vi "ExStreamToFilefNoDisplay.vi"() -> ()   [LabVIEW 2010]
uses:
  Open-Close Hardware/CamHandle.vi
panel:
  out "done collecting":bool
  out "beta":u32
  out "build":u32
  out "Minor":u32
  out "Major":u32
  in  "stop collection 2":bool
  in  "data collection type\n1 - stream to file\n2 - stream to ram, then file":u32=2 min=1 step=1
  in  "stop collection":bool
  in  "Path":path=path "C:/Users/Public/Documents/SItoolkit/LabVIEW/Data Files/nframe"
  in  "Number of Images":u32=50 min=1 step=1
  out "ready to \nstart":bool
  in  "Start collection":bool
  in  "Exposure":dbl=1e-05 min=0.0 step=1e-06 format="%.7f"
  out "error out":errorcluster
  in  "error in (no error)":errorcluster
  # "ExCNframeBigBufNoDisplay:\nThis example collects,  and saves in \na .spe file the number of images selected. This \nexample requires the camera have circular \nbuffers capability. \nFirst this example creates an array of image \nhandles. It then collects data into this array.\nFinally it displays and saves all the images."
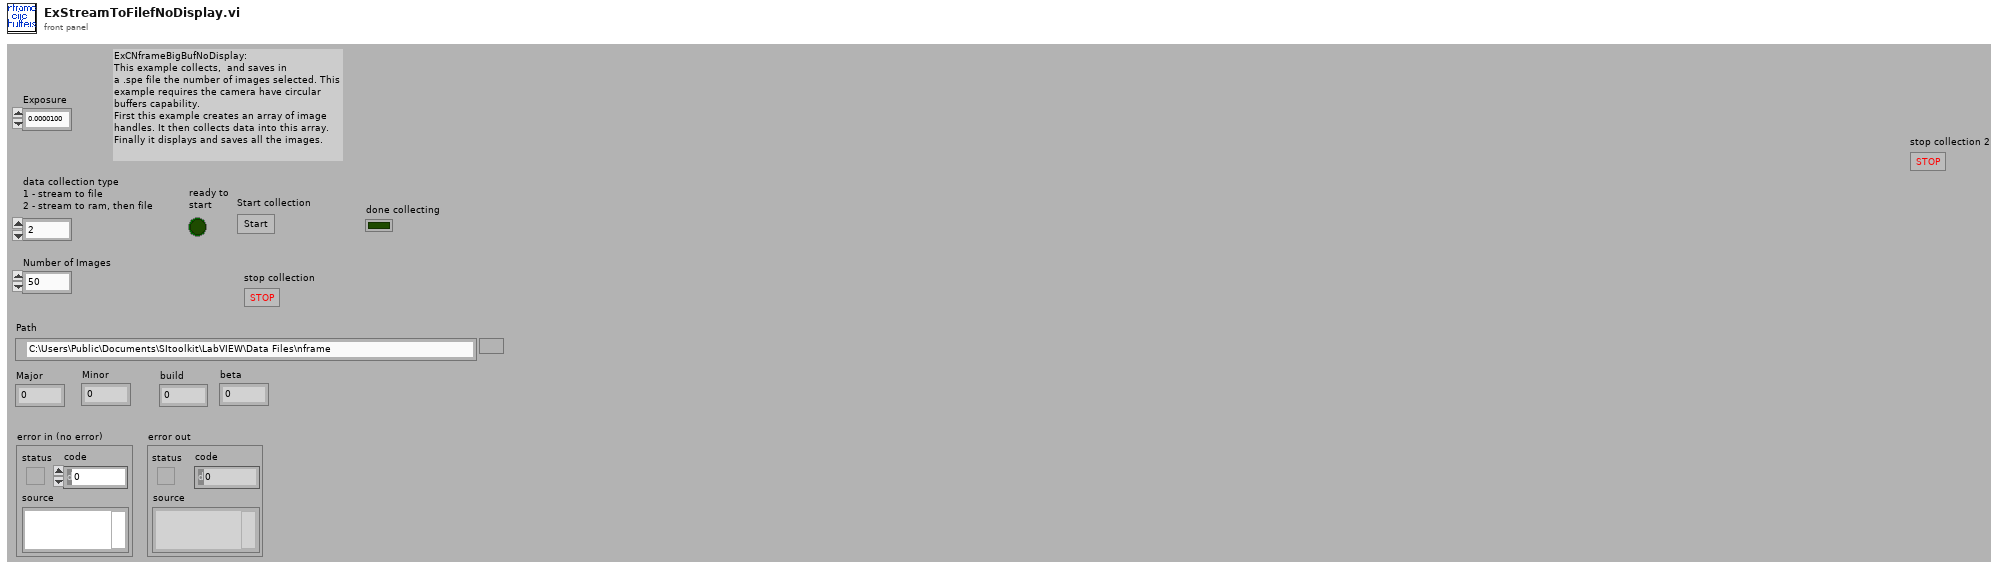
[diagram p1: front panel]
types:
  T1 = cluster{"Major Version":u32, "Minor Version":u32, "External Build":u32, "Internal Build":u32}
  T2 = cluster{"acquire focus mode":u32, "Exposure":dbl, "Number of Images":u32, "Software accumulation":u32}
  T3 = cluster{"Camera Handle":u32, "Pulser Handle":u32, "File Handle":u32, "Display Handle":u32, "Image Handle":u32}
  T4 = cluster{"Exposure":dbl, "acquire focus mode":u32, "Number of Images":u32, "Software accumulation":u32}
  T5 = cluster{"Camera Handle":u32, "File Handle":u32, "Image Handle":u32}
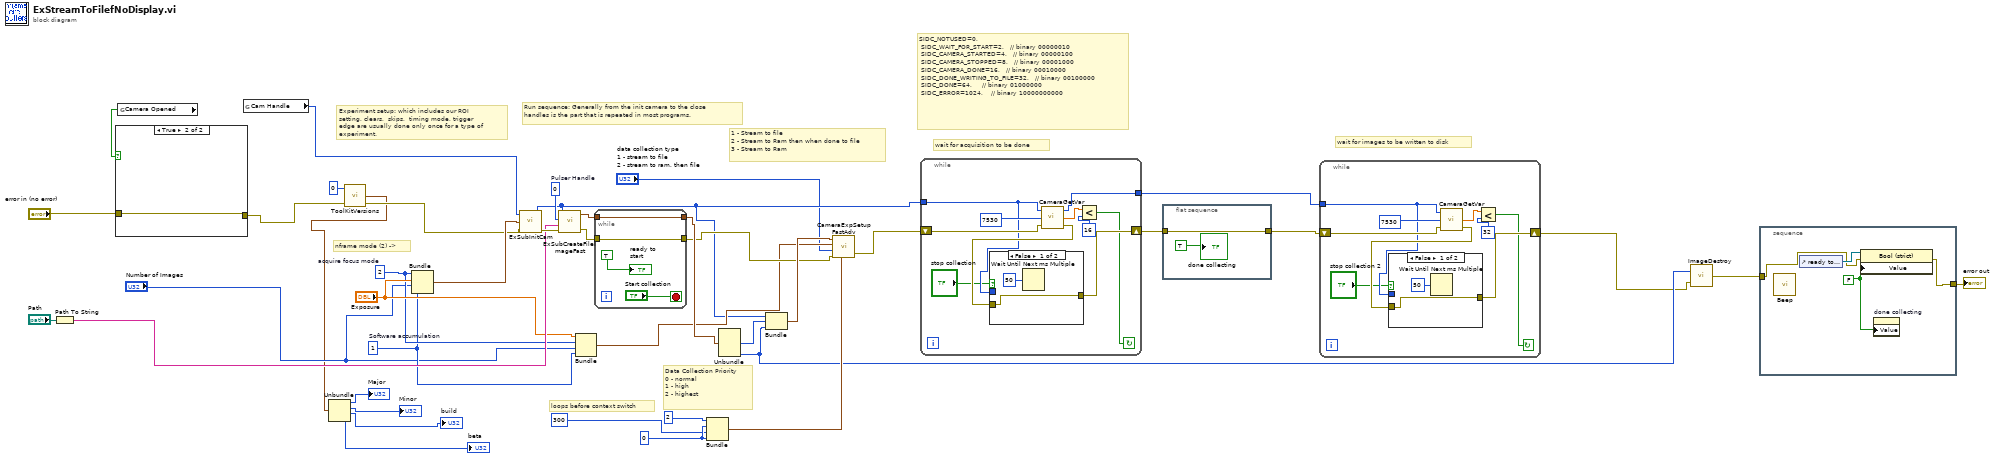
[diagram p0: block diagram]
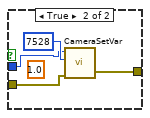
[diagram p2: hidden frame]
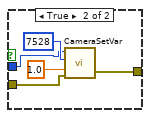
[diagram p3: hidden frame]
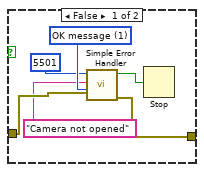
[diagram p4: hidden frame]
diagram:
  w29 = u32 0
  w40 = u32 0  # Pulser Handle
  w26 = u32 2  # acquire focus mode
  w25 = u32 1  # Software accumulation
  # "SIDC_NOTUSED=0,\n\tSIDC_WAIT_FOR_START=2,\t\t\t// binary 00000010\n\tSIDC_CAMERA_STARTED=4,\t\t\t// binary 00000100\n\tSIDC_CAMERA_STOPPED=8,\t\t\t// binary 00001000\n\tSIDC_CAMERA_DONE=16,\t\t\t// binary 00010000\n\tSIDC_DONE_WRITING_TO_FILE=32,   // binary 00100000\n\tSIDC_DONE=64,\t\t\t\t\t// binary 01000000\n\tSIDC_ERROR=1024,\t\t\t\t// binary 10000000000"
  # "wait for images to be written to disk"
  # "wait for acquisition to be done"
  # "loops before context switch"
  # "Data Collection Priority\n0 - normal\n1 - high\n2 - highest"
  # "1 - Stream to file\n2 - Stream to Ram then when done to file\n3 - Stream to Ram"
  # "Run sequence: Generally from the init camera to the close \nhandles is the part that is repeated in most programs."
  # "Experiment setup: which includes our ROI setting, clears,  skips,  timing mode, trigger edge are usually done only once for a type of experiment."
  # "nframe mode (2) ->"
  n1 = Path To String(path="Path") -> (string=w33:string)
  n2 = global read "CamHandle.vi" "Camera Opened"() -> (w36:bool)
  n3 = case shown="True" w36 {
    tunnel: "error in (no error)" -> [w46 w48]
    tunnel: [w45 w48] -> w9
    frame False {
      w47 = u16 1 items=["no dialog", "OK message", "continue or stop message"] ("type of dialog (OK msg:1)")
      n4 = call <vilib>:"Simple Error Handler.vi"("error code (no error:0)"=5501, "error source (\" \")"="Camera not opened", "type of dialog (OK msg:1)"=w47, "error in (no error)"=w46) -> ("error?"=w43:bool, "error out"=w45:errorcluster)  [unwired: 1 in, 3 out]
      n5 = Stop(stop? (T)=w43) -> ()
    }
    frame True {
    }
  }
  n6 = global read "CamHandle.vi" "Cam Handle"() -> (w12:u32)
  n7 = call <userlib>:"ToolKitVersions.vi"("error in"=w9, "Index"=u32 0) -> ("error out"=w10:errorcluster, "Versions"=w8:T1)  [unwired: 1 in, 1 out]
  n8 = Unbundle(w8) -> ("Major Version"=→"Major":u32, "Minor Version"=→"Minor":u32, "External Build"=→"build":u32, "Internal Build"=→"beta":u32)
  n9 = Bundle("acquire focus mode"=w26, "Exposure"="Exposure", "Number of Images"="Number of Images", "Software accumulation"=w25) -> (w21:T2)  [unwired: 1 in]
  n10 = call "ExSubInitCam.vi"("error in (no error)"=w10, "Camera Information"=w21, "Camera Handle"=w12) -> ("error out"=w41:errorcluster, "Camera Handle"=w16:u32)
  n11 = call "ExSubCreateFileImageFast.vi"("Camera Handle"=w16, "Pulser Handle"=w40, "File and Display Name"=w33, "error in (no error)"=w41) -> ("Handles Out"=w39:T3, "error out"=w38:errorcluster)  [unwired: 2 in]
  n12 = Bundle("Exposure"="Exposure", "acquire focus mode"=w26, "Number of Images"="Number of Images", "Software accumulation"=w25) -> (w23:T4)  [unwired: 1 in]
  n13 = while {
    tunnel: w39 -> [w52]
    tunnel: [w52] -> w32
    tunnel: w38 -> [w51]
    tunnel: [w51] -> w24
    stop <- "Start collection" stop-if-true
    "ready to \nstart" <- TRUE
  }
  n14 = Bundle(u32 2, w29, 300, w29) -> (w28:cluster{u32, u32, i32, u32})  [unwired: 1 in]
  n15 = Unbundle(w32) -> ("File Handle"=w20:u32, "Image Handle"=w17:u32)  [unwired: 3 out]
  n16 = Bundle("Camera Handle"=w16, "File Handle"=w20, "Image Handle"=w17) -> (w31:T5)  [unwired: 1 in]
  n17 = call <userlib>:"CameraExpSetupFastAdv.vi"("Handles In"=w31, "Experiment Setup"=w23, "Type Of Collection"="data collection type\n1 - stream to file\n2 - stream to ram, then file", "error in (no error)"=w24, "Thread Control"=w28) -> ("error out"=w19:errorcluster)  [unwired: 1 out]
  n18 = while {
    shift-right: [w59] -> w3
    shift-left: w19 -> [w61]
    tunnel: w16 -> [w58]
    tunnel: [w53] -> w13
    stop <- w54 continue-if-true
    n19 = call <userlib>:"CameraGetVar.vi"("error in"=w61, "Parameter ID"=7530, "Camera Handle"=w58) -> ("error out"=w60:errorcluster, "Value"=w56:dbl, "Camera Handle"=w53:u32)
    n20 = case shown="False" "stop collection" {
      tunnel: w60 -> [w64 w68]
      tunnel: [w64 w67] -> w59
      tunnel: w58 -> [_ w66]
      frame False {
        n21 = Wait Until Next ms Multiple(millisecond multiple=u32 50) -> ()  [unwired: 1 out]
      }
      frame True {
        n22 = call <userlib>:"CameraSetVar.vi"("error in"=w68, "Value"=1.0, "Parameter ID"=7528, "Camera Handle"=w66) -> ("error out"=w67:errorcluster)  [unwired: 1 out]
      }
    }
    n23 = Less?(x=w56, y=16) -> (x < y?=w54:bool)
  }
  n24 = flat-sequence {
    tunnel: w3 -> [w71]
    tunnel: [w71] -> w2
    frame #0 {
      "done collecting" <- TRUE
    }
  }
  n25 = while {
    shift-right: [w77] -> w1
    shift-left: w2 -> [w79]
    tunnel: w13 -> [w76]
    stop <- w72 continue-if-true
    n26 = call <userlib>:"CameraGetVar.vi"("error in"=w79, "Parameter ID"=7530, "Camera Handle"=w76) -> ("error out"=w78:errorcluster, "Value"=w74:dbl)  [unwired: 1 out]
    n27 = case shown="False" "stop collection 2" {
      tunnel: w78 -> [w82 w85]
      tunnel: [w82 w84] -> w77
      tunnel: w76 -> [_ w83]
      frame False {
        n28 = Wait Until Next ms Multiple(millisecond multiple=u32 50) -> ()  [unwired: 1 out]
      }
      frame True {
        (unwired) 1.0
        n29 = call <userlib>:"CameraSetVar.vi"("error in"=w85, "Parameter ID"=7528, "Camera Handle"=w83) -> ("error out"=w84:errorcluster)  [unwired: 1 in, 1 out]
      }
    }
    n30 = Less?(x=w74, y=32) -> (x < y?=w72:bool)
  }
  n31 = call <userlib>:"ImageDestroy.vi"("error in"=w1, "Data handle"=w17) -> ("error out"=w18:errorcluster)
  n32 = stacked-sequence {
    tunnel: [w89] -> w35
    tunnel: w18 -> [w88]
    frame #0 {
      w87 = FALSE
      n33 = call <vilib>:"Beep.vi"() -> ()  [unwired: 12 in]
      n34 = control-ref of="ready to \nstart"() -> (w90:refnum<vi>)
      n35 = property class="Bool (strict)"(reference=w90, error in=w88, "Value"=w87) -> (error out=w89:errorcluster)  [unwired: 1 out]
      n36 = property on="done collecting" class="Bool (strict)"("Value"=w87) -> ()  [unwired: 2 in, 2 out]
    }
  }
  "error out" <- w35
